vi "Util Byte Array to Hex String.vi"(8 "error in (no error)":errorcluster, 11 "Byte Array":u8[](array[numeric]) format="%x") -> (0 "error out":errorcluster, 3 "Hex String":string)   [LabVIEW 2017, in "xHelper.lvlib"]
uses:
  xHelper.lvlib
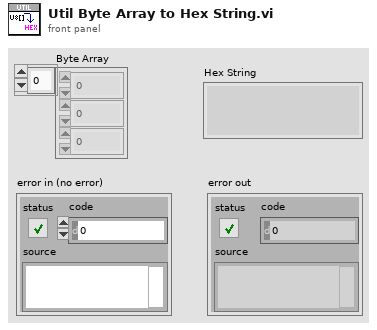
[diagram p1: front panel]
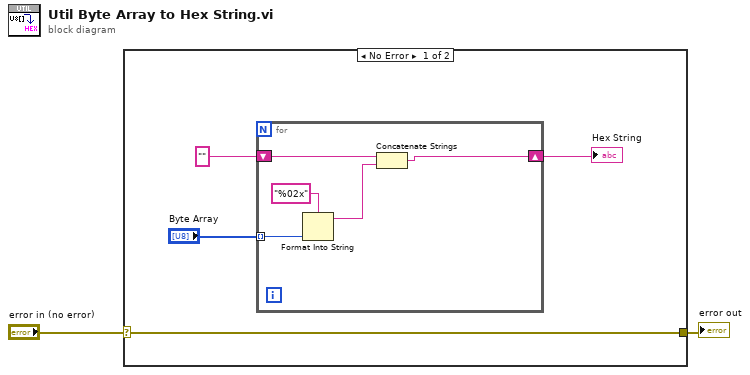
[diagram p0: block diagram]
diagram:
  n1 = case shown="No Error" "error in (no error)" {
    selector: "error in (no error)" -> [w3 w12]
    tunnel: [w3 w12] -> w1
    frame No Error {
      n2 = for {
        tunnel: "Byte Array" -> [w11] mode=indexing
        shift-right: [w8] -> w4
        shift-left: "" -> [w9]
        n3 = Format Into String(format string="%02x", w11) -> (resulting string=w7:string)  [unwired: 2 in, 1 out]
        n4 = Concatenate Strings(w9, w7) -> (w8:string)
      }
      "Hex String" <- w4
    }
    frame Error {
    }
  }
  "error out" <- w1
